vi "Reverse Configurations for Safe PowerDown.vi"(0 "Data Cluster":T1={"session reservation"=refnum, "measurement context"=refnum, "Measurement Configuration"={"Quick Power Down"=FALSE, "Pin Name"=[], "Source Mode"=[], "Start Value"=[], "Target Value"=[], "Compliance Limit"=[], "Sense Mode"=[], "Default Ramp Rate"=[], "Ramp Rate"=[], "Start Delay"=[], "Relative To"=[], "Transient Response"=[], "Data Capture"=FALSE, "Power line frequency"=1}, "Measurement Results"={"Voltage Measurements"=[], "Current Measurements"=[], "Indices"=[], "dt values"=[], "Default Ramp Rate?"=[], "Actual Ramp Rates"=[], "Warning"=[], "Operation Complete?"=FALSE}, "Channel Settings"={"Channel Name"=[], "Channel Number"=[], "Instrument handle"=[], "Session Exists?"=[], "Session.name"=[]}, "Software Flags"={"Initialize Complete?"=FALSE, "Configuration Complete?"=FALSE, "Run Complete?"=FALSE, "Output Complete?"=FALSE, "Safe Power Down In Progress?"=FALSE, "Power Up Operation?"=FALSE, "Canceled?"=FALSE, "Session exists?"=[], "Advanced Seq Created?"=[], "Initiated?"=[], "Unsupported Ramp?"=[], "Compliance Reached?"=[], "PowerUp?"=FALSE, "Unsupported Start Delay?"=[]}, "Ramp Configurations"={"Minimum Sequence dt(s)"=[], "Sequence Delta(s)"=[], "Number of steps"=[], "Actual Ramp Rate(Unit/S)"=[], "Total Sequence Time"=0.0, "Rising Period"=[], "Accumulative Start Delay(s)"=[], "Temporary Target Level"=[], "Start Level"=[], "Measure Period"=0.0, "Compliance Skip Duration"=[], "Max Sequence Period Index"=0, "Compliance Check Duration"=0.0}, "Error Info"={"Error Occurred?"=FALSE, "Warning List"=[], "Error Phase"="", "Error Code"=5100, "error"={"status"=FALSE, "code"=0, "source"=""}, "Error List"=[], "Custom Error?"=FALSE}, "Measurements"={"Measurements"=[], "Calculated Ramp Rate"=[], "Default RampRate?"=[], "Aperture Time"=[]}, "Log"={"User Event"=refnum, "Measure Complete"=FALSE, "Log File Ref."=refnum, "Log Data?"=FALSE, "Async Log Ref."=refnum}} {"Measurement Configuration"."Relative To" items=["Power sequence start", "Previous source start", "Previous source end"]; "Measurement Configuration"."Power line frequency" items=["50 Hz", "60 Hz"]; "Measurement Configuration"."Start Value" format="%#_6p"; "Measurement Configuration"."Transient Response" items=["Slow", "Normal", "Fast"]; "Measurement Configuration"."Sense Mode" items=["Local Sense", "Remote Sense"]; "Measurement Configuration"."Target Value" format="%#_6p"; "Measurement Configuration"."Source Mode" items=["DC Voltage", "DC Current"]; "Measurement Configuration"."Start Delay" format="%#_6p"; "Measurement Configuration"."Compliance Limit" format="%#_6p"; "Measurement Configuration"."Ramp Rate" format="%#_6p"}, 11 "error in (no error)":errorcluster) -> (4 "Data Cluster OUT":T1={"session reservation"=refnum, "measurement context"=refnum, "Measurement Configuration"={"Quick Power Down"=FALSE, "Pin Name"=[], "Source Mode"=[], "Start Value"=[], "Target Value"=[], "Compliance Limit"=[], "Sense Mode"=[], "Default Ramp Rate"=[], "Ramp Rate"=[], "Start Delay"=[], "Relative To"=[], "Transient Response"=[], "Data Capture"=FALSE, "Power line frequency"=1}, "Measurement Results"={"Voltage Measurements"=[], "Current Measurements"=[], "Indices"=[], "dt values"=[], "Default Ramp Rate?"=[], "Actual Ramp Rates"=[], "Warning"=[], "Operation Complete?"=FALSE}, "Channel Settings"={"Channel Name"=[], "Channel Number"=[], "Instrument handle"=[], "Session Exists?"=[], "Session.name"=[]}, "Software Flags"={"Initialize Complete?"=FALSE, "Configuration Complete?"=FALSE, "Run Complete?"=FALSE, "Output Complete?"=FALSE, "Safe Power Down In Progress?"=FALSE, "Power Up Operation?"=FALSE, "Canceled?"=FALSE, "Session exists?"=[], "Advanced Seq Created?"=[], "Initiated?"=[], "Unsupported Ramp?"=[], "Compliance Reached?"=[], "PowerUp?"=FALSE, "Unsupported Start Delay?"=[]}, "Ramp Configurations"={"Minimum Sequence dt(s)"=[], "Sequence Delta(s)"=[], "Number of steps"=[], "Actual Ramp Rate(Unit/S)"=[], "Total Sequence Time"=0.0, "Rising Period"=[], "Accumulative Start Delay(s)"=[], "Temporary Target Level"=[], "Start Level"=[], "Measure Period"=0.0, "Compliance Skip Duration"=[], "Max Sequence Period Index"=0, "Compliance Check Duration"=0.0}, "Error Info"={"Error Occurred?"=FALSE, "Warning List"=[], "Error Phase"="", "Error Code"=5100, "error"={"status"=FALSE, "code"=0, "source"=""}, "Error List"=[], "Custom Error?"=FALSE}, "Measurements"={"Measurements"=[], "Calculated Ramp Rate"=[], "Default RampRate?"=[], "Aperture Time"=[]}, "Log"={"User Event"=refnum, "Measure Complete"=FALSE, "Log File Ref."=refnum, "Log Data?"=FALSE, "Async Log Ref."=refnum}} {"Measurement Configuration"."Relative To" items=["Power sequence start", "Previous source start", "Previous source end"]; "Measurement Configuration"."Power line frequency" items=["50 Hz", "60 Hz"]; "Measurement Configuration"."Start Value" format="%#_6p"; "Measurement Configuration"."Transient Response" items=["Slow", "Normal", "Fast"]; "Measurement Configuration"."Sense Mode" items=["Local Sense", "Remote Sense"]; "Measurement Configuration"."Target Value" format="%#_6p"; "Measurement Configuration"."Source Mode" items=["DC Voltage", "DC Current"]; "Measurement Configuration"."Start Delay" format="%#_6p"; "Measurement Configuration"."Compliance Limit" format="%#_6p"; "Measurement Configuration"."Ramp Rate" format="%#_6p"}, 15 "error out":errorcluster)   [LabVIEW 2024, in "devicePowerSequencerCoreLogic.lvlib"]
uses:
  devicePowerSequencerCoreLogic.lvlib
  controls/Data Cluster.ctl
  <vilib>/Plug-In SDKs/Clients/Session Management V1/Session Reservation/Session Reservation.lvclass
  <vilib>/Plug-In SDKs/Measurements/Measure Call Context/Measure Call Context.lvclass
  Measurement Configuration.ctl
  controls/Source Mode.ctl
  controls/Sense Mode.ctl
  controls/Relative To.ctl
  controls/Transient Response.ctl
  controls/Power line frequency.ctl
  Measurement Results.ctl
  controls/Channel Name.ctl
  controls/Software Flags.ctl
  controls/Ramp Configurations.ctl
  controls/Error Info.ctl
  controls/Measurements.ctl
  controls/Voltage and Current Measurements.ctl
  controls/Log Configurations.ctl
  Device Power Sequencer.lvlib
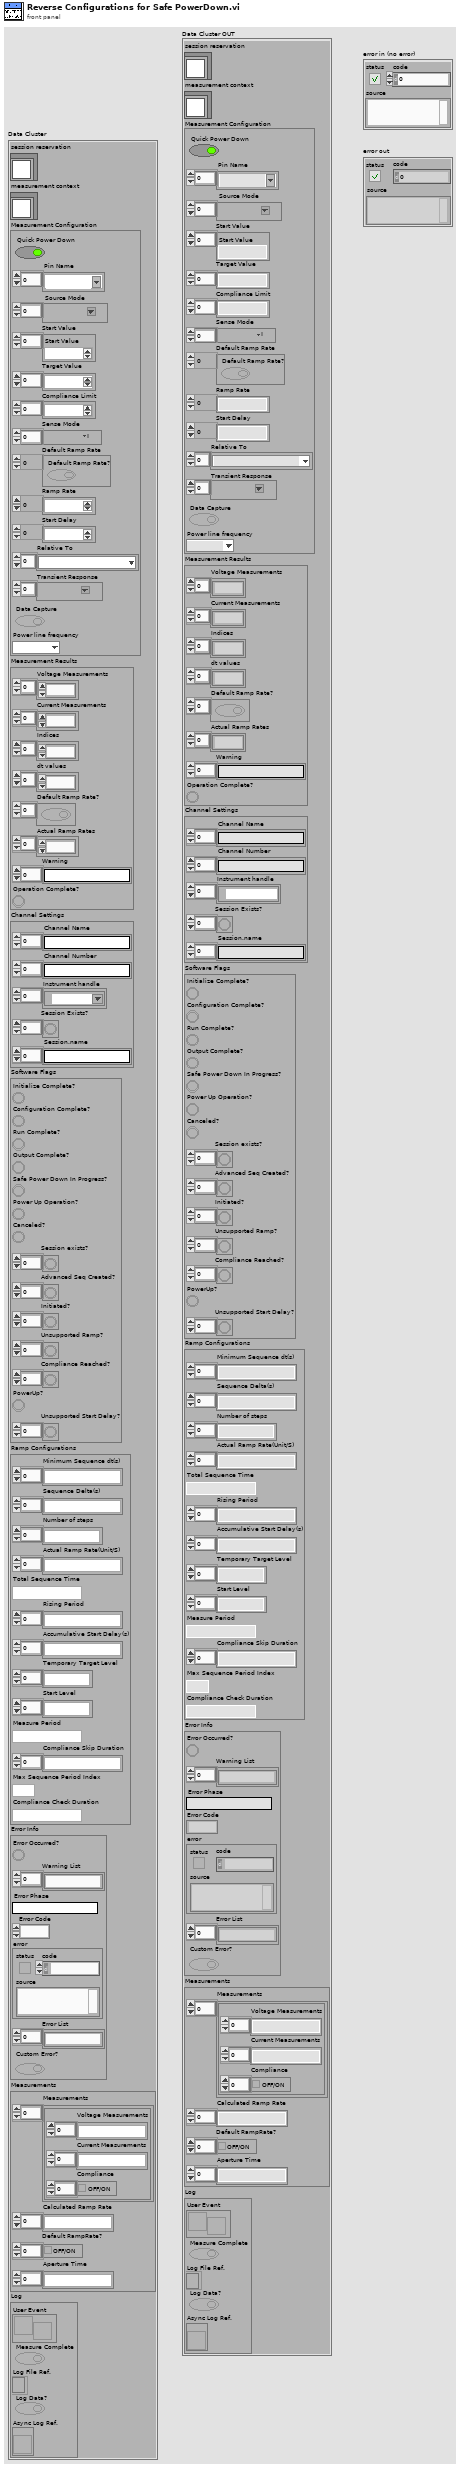
[diagram p1: front panel]
types:
  T1 = typedef "devicePowerSequencerCoreLogic.lvlib/Data Cluster.ctl" = cluster{"session reservation":refnum<class "Session Reservation.lvclass">, "measurement context":refnum<class "Measure Call Context.lvclass">, "Measurement Configuration":T2, "Measurement Results":T8, "Channel Settings":T9, "Software Flags":T10, "Ramp Configurations":T11, "Error Info":T12, "Measurements":T13, "Log":T15}
  T2 = typedef "Device Power Sequencer.lvlib/Measurement Configuration.ctl" = cluster{"Quick Power Down":bool, "Pin Name":string[], "Source Mode":T3[], "Start Value":dbl[], "Target Value":dbl[], "Compliance Limit":dbl[], "Sense Mode":T4[], "Default Ramp Rate":bool[], "Ramp Rate":dbl[], "Start Delay":dbl[], "Relative To":T5[], "Transient Response":T6[], "Data Capture":bool, "Power line frequency":T7}
  T3 = typedef "Device Power Sequencer.lvlib/Source Mode.ctl" = i32
  T4 = typedef "Device Power Sequencer.lvlib/Sense Mode.ctl" = i32
  T5 = typedef "Device Power Sequencer.lvlib/Relative To.ctl" = u32
  T6 = typedef "Device Power Sequencer.lvlib/Transient Response.ctl" = i32
  T7 = typedef "Device Power Sequencer.lvlib/Power line frequency.ctl" = u32
  T8 = typedef "Device Power Sequencer.lvlib/Measurement Results.ctl" = cluster{"Voltage Measurements":dbl[], "Current Measurements":dbl[], "Indices":i32[], "dt values":dbl[], "Default Ramp Rate?":bool[], "Actual Ramp Rates":dbl[], "Warning":string[], "Operation Complete?":bool}
  T9 = typedef "devicePowerSequencerCoreLogic.lvlib/Channel Name.ctl" = cluster{"Channel Name":string[], "Channel Number":string[], "Instrument handle":refnum<k15>[], "Session Exists?":bool[], "Session.name":string[]}
  T10 = typedef "devicePowerSequencerCoreLogic.lvlib/Software Flags.ctl" = cluster{"Initialize Complete?":bool, "Configuration Complete?":bool, "Run Complete?":bool, "Output Complete?":bool, "Safe Power Down In Progress?":bool, "Power Up Operation?":bool, "Canceled?":bool, "Session exists?":bool[], "Advanced Seq Created?":bool[], "Initiated?":bool[], "Unsupported Ramp?":bool[], "Compliance Reached?":bool[], "PowerUp?":bool, "Unsupported Start Delay?":bool[]}
  T11 = typedef "devicePowerSequencerCoreLogic.lvlib/Ramp Configurations.ctl" = cluster{"Minimum Sequence dt(s)":dbl[], "Sequence Delta(s)":dbl[], "Number of steps":i32[], "Actual Ramp Rate(Unit/S)":dbl[], "Total Sequence Time":dbl, "Rising Period":dbl[], "Accumulative Start Delay(s)":dbl[], "Temporary Target Level":dbl[], "Start Level":dbl[], "Measure Period":dbl, "Compliance Skip Duration":dbl[], "Max Sequence Period Index":i32, "Compliance Check Duration":dbl}
  T12 = typedef "devicePowerSequencerCoreLogic.lvlib/Error Info.ctl" = cluster{"Error Occurred?":bool, "Warning List":string[], "Error Phase":string, "Error Code":i32, "error":errorcluster, "Error List":string[], "Custom Error?":bool}
  T13 = typedef "devicePowerSequencerCoreLogic.lvlib/Measurements.ctl" = cluster{"Measurements":T14[], "Calculated Ramp Rate":dbl[], "Default RampRate?":bool[], "Aperture Time":dbl[]}
  T14 = typedef "devicePowerSequencerCoreLogic.lvlib/Voltage and Current Measurements.ctl" = cluster{"Voltage Measurements":dbl[], "Current Measurements":dbl[], "Compliance":bool[]}
  T15 = typedef "devicePowerSequencerCoreLogic.lvlib/Log Configurations.ctl" = cluster{"User Event":refnum<user-event>, "Measure Complete":bool, "Log File Ref.":refnum<file>, "Log Data?":bool, "Async Log Ref.":refnum<vi>}
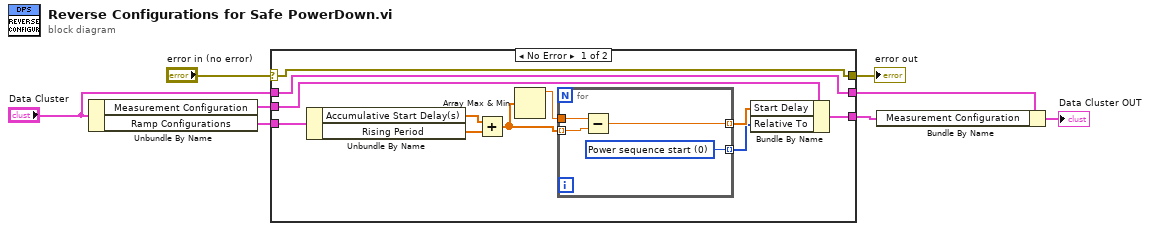
[diagram p0: block diagram]
diagram:
  n1 = Unbundle By Name("Data Cluster") -> ("Measurement Configuration"=w6:T2, "Ramp Configurations"=w5:T11)
  n2 = case shown="No Error" "error in (no error)" {
    selector: "error in (no error)" -> [w17 w25]
    tunnel: w6 -> [w19 w26]
    tunnel: [w18 w26] -> w2
    tunnel: [w17 w25] -> w7
    tunnel: w5 -> [w16 _]
    tunnel: "Data Cluster" -> [w15 w24]
    tunnel: [w15 w24] -> w3
    frame No Error {
      n3 = Unbundle By Name(w16) -> ("Accumulative Start Delay(s)"=w14:dbl[], "Rising Period"=w9:dbl[])
      n4 = Add(x=w14, y=w9) -> (x+y=w10:dbl[])
      n5 = Array Max & Min(array=w10) -> (max value=w13:dbl)  [unwired: 3 out]
      n6 = for {
        tunnel: w10 -> [w23] mode=indexing
        tunnel: w13 -> [w22]
        tunnel: [w21] -> w12 mode=indexing
        tunnel: [w20] -> w11 mode=indexing
        w20 = T5 0 items=["Power sequence start", "Previous source start", "Previous source end"] ("Relative To")
        n7 = Subtract(x=w22, y=w23) -> (x-y=w21:dbl)
      }
      n8 = Bundle By Name(cluster=w19, "Start Delay"=w12, "Relative To"=w11) -> (w18:T2)
    }
    frame Error {
    }
  }
  "error out" <- w7
  n9 = Bundle By Name(cluster=w3, "Measurement Configuration"=w2) -> (→"Data Cluster OUT":T1)
